vi "Pcre2Substitute8.vi"(0 "pCode":u64 format="%.0x", 1 "Options":u32 format="%.0x", 3 "pMatchContext":u64 format="%.0x", 5 "Subject":string, 7 "Replacement":string, 9 "StartOffset":u64, 11 "error in":errorcluster, 12 "pMatchData":u64 format="%.0x") -> (4 "pCode":u64 format="%.0x", 6 "OutString":string, 14 "pMatchData":u64 format="%.0x", 15 "error out":errorcluster)   [LabVIEW 2021, in "libpcre2-8.lvlib"]
uses:
  libpcre2-8.lvlib
  libpcre2-8-x32.dll
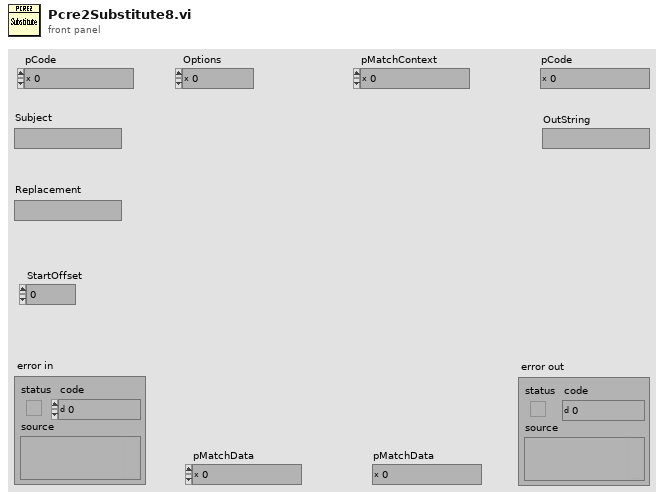
[diagram p1: front panel]
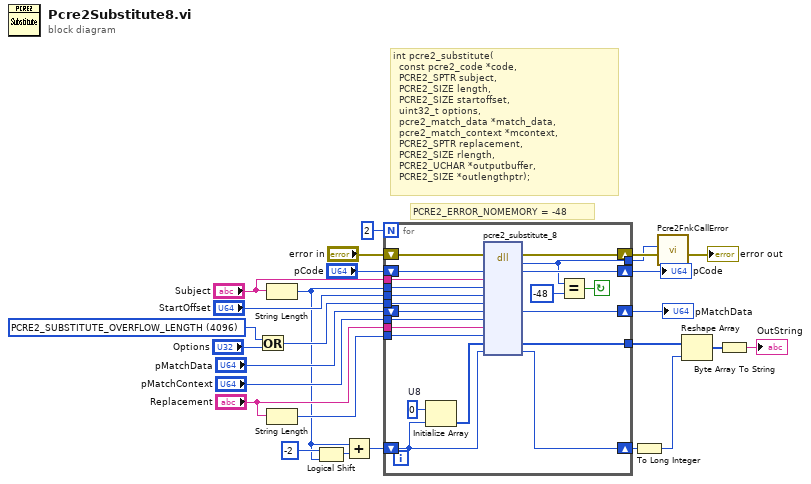
[diagram p0: block diagram]
diagram:
  w9 = u32 4096 items=["PCRE2_NOOPTION"=0, "PCRE2_NOTBOL"=1, "PCRE2_NOTEOL"=2, "PCRE2_NOTEMPTY"=4, "PCRE2_NOTEMPTY_ATSTART"=8, "PCRE2_PARTIAL_SOFT"=16, "PCRE2_PARTIAL_HARD"=32, "PCRE2_DFA_RESTART"=64, "PCRE2_DFA_SHORTEST"=128, "PCRE2_SUBSTITUTE_GLOBAL"=256, "PCRE2_SUBSTITUTE_EXTENDED"=512, "PCRE2_SUBSTITUTE_UNSET_EMPTY"=1024, "PCRE2_SUBSTITUTE_UNKNOWN_UNSET"=2048, "PCRE2_SUBSTITUTE_OVERFLOW_LENGTH"=4096, "PCRE2_NO_JIT"=8192, "PCRE2_COPY_MATCHED_SUBJECT"=16384, "PCRE2_SUBSTITUTE_LITERAL"=32768, "PCRE2_SUBSTITUTE_MATCHED"=65536, "PCRE2_SUBSTITUTE_REPLACEMENT_ONLY"=131072, "PCRE2_DISABLE_RECURSELOOP_CHECK"=262144, "PCRE2_ENDANCHORED"=536870912, "PCRE2_NO_UTF_CHECK"=1073741824, "PCRE2_ANCHORED"=2147483648] ("MatchOption")
  # "PCRE2_ERROR_NOMEMORY = -48"
  # "int pcre2_substitute(\n  const pcre2_code *code,\n  PCRE2_SPTR subject,\n  PCRE2_SIZE length,\n  PCRE2_SIZE startoffset,\n  uint32_t options,\n  pcre2_match_data *match_data,\n  pcre2_match_context *mcontext,\n  PCRE2_SPTR replacement,\n  PCRE2_SIZE rlength,\n  PCRE2_UCHAR *outputbuffer,\n  PCRE2_SIZE *outlengthptr);"
  n1 = Or(x=w9, y="Options") -> (x .or. y?=w13:u32)
  n2 = String Length(string="Subject") -> (length=w11:i32)
  n3 = String Length(string="Replacement") -> (length=w16:i32)
  n4 = Logical Shift(y=i16 -2, x=w11) -> (x << y=w12:i32)
  n5 = Add(x=w11, y=w12) -> (x+y=w6:i32)
  n6 = for {
    N: 2 -> [_]
    tunnel: "StartOffset" -> [w47]
    tunnel: "pMatchContext" -> [w44]
    tunnel: "Replacement" -> [w39]
    tunnel: w16 -> [w38]
    tunnel: "Subject" -> [w37]
    tunnel: w13 -> [w36]
    tunnel: w11 -> [w35]
    tunnel: [w33] -> w8
    shift-right: [w45] -> w23
    shift-left: "error in" -> [w46]
    shift-right: [w41] -> w19
    shift-left: "pCode" -> [w42]
    shift-right: [w40] -> w18
    shift-left: "pMatchData" -> [w43]
    shift-right: [w30] -> w4
    shift-left: w6 -> [w27]
    tunnel: [w29] -> w5
    stop <- w31 continue-if-true
    w28 = u8 0  # U8
    n7 = Initialize Array(w28, w27) -> (w34:u8[])
    n8 = dll-call lib="libpcre2-8-x*.dll" fn="pcre2_substitute_8"(error in=w46, "code"=w42, "subject"=w37, "length"=w35, "startoffset"=w47, "options"=w36, "match_data"=w43, "mcontext"=w44, "replacement"=w39, "rlength"=w38, "outbuffer"=w34, "outlengthptr"=w27) -> (error out=w45:errorcluster, "result"=w33:i32, "code"=w41:u64, "match_data"=w40:u64, "outbuffer"=w29:u8[], "outlengthptr"=w30:u64)  [unwired: 9 in, 1 out]
    n9 = Equal?(x=w33, y=-48) -> (x = y?=w31:bool)
  }
  "pCode" <- w19
  "pMatchData" <- w18
  n10 = To Long Integer(number=w4) -> (32bit integer=w3:i32)
  n11 = call "Pcre2FnkCallError.vi"("error in"=w23, "ErrorCode"=w8) -> ("error out"=→"error out":errorcluster)  [unwired: 9 in]
  n12 = Reshape Array(w5, w3) -> (w2:u8[])
  n13 = Byte Array To String(unsigned byte array=w2) -> (string=→"OutString":string)
